vi "Register gRPC Methods.vi"(8 "error in (no error)":errorcluster, 11 "Template Server in":refnum<class "MicronGRPC.lvclass">) -> (0 "error out":errorcluster, 3 "Template Server out":refnum<class "MicronGRPC.lvclass">)   [LabVIEW 2019, in "MicronGRPCGeneratedServer.lvlib" / "MicronGRPC.lvclass"]
uses:
  MicronGRPC.lvclass
  typeDefs/Server Internal UEs.ctl
  typeDefs/Server Internal Message.ctl
  typeDefs/Server gRPC UEs.ctl
  <vilib>/gRPC/LabVIEW gRPC Library/Server API/typeDefs/gRPCId Cluster.ctl
  <vilib>/gRPC/LabVIEW gRPC Library/Shared/grpcId.ctl
  MicronGRPC.lvclass/MicronGRPC.ctl
  <vilib>/gRPC/LabVIEW gRPC Library/grpc-lvsupport-release.lvlib
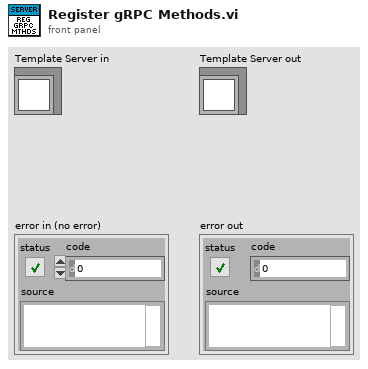
[diagram p1: front panel]
types:
  T1 = typedef "MicronGRPCGeneratedServer.lvlib/MicronGRPC.lvclass/Server gRPC UEs.ctl" = cluster{"MicronGRPC Message gRPC UE":refnum<user-event>}
  T2 = typedef "MicronGRPCGeneratedServer.lvlib/MicronGRPC.lvclass/Server Internal UEs.ctl" = cluster{"MicronGRPC Message Internal UE":refnum<user-event>}
  T3 = typedef "grpc-lvsupport-release.lvlib/grpcId.ctl" = u64
  T4 = typedef "MicronGRPCGeneratedServer.lvlib/MicronGRPC.lvclass/Server Internal Message UE.ctl" = refnum<user-event>
  T5 = typedef "grpc-lvsupport-release.lvlib/gRPCId Cluster UE.ctl" = refnum<user-event>
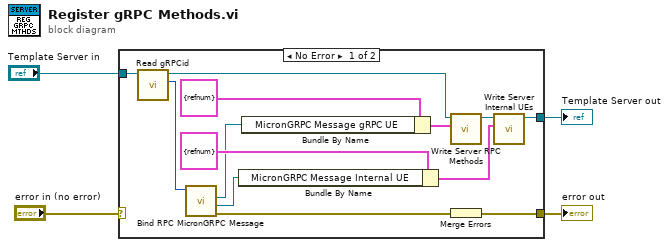
[diagram p0: block diagram]
diagram:
  n1 = case shown="No Error" "error in (no error)" {
    selector: "error in (no error)" -> [_ w18]
    tunnel: "Template Server in" -> [w9 w19]
    tunnel: [w17 w18] -> w3
    tunnel: [w16 w19] -> w2
    frame No Error {
      n2 = call-dynamic "Read gRPCid.vi"("gRPC service in"=w9) -> ("gRPCid"=w8:T3, "gRPC service out"=w10:refnum<class "MicronGRPC.lvclass">)  [unwired: 8 in, 1 out]
      n3 = call "Bind RPC MicronGRPC Message.vi"("gRPCid server in"=w8) -> ("error out"=w7:errorcluster, "MicronGRPC Message Internal UE"=w6:T4, "MicronGRPC Message gRPC UE"=w5:T5)  [unwired: 7 in, 1 out]
      n4 = Bundle By Name ("Bundle Internal UEs")(cluster=T2 {"MicronGRPC Message Internal UE"=refnum} ("Server Internal UEs"), "MicronGRPC Message Internal UE"=w6) -> (w15:T2)
      n5 = Bundle By Name ("Bundle gRPC UEs")(cluster=T1 {"MicronGRPC Message gRPC UE"=refnum} ("gRPC Server Method Events"), "MicronGRPC Message gRPC UE"=w5) -> (w12:T1)
      n6 = call "Write Server RPC Methods.vi"("Server RPC Methods"=w12, "SignalGeneratorService in"=w10) -> ("SignalGeneratorService out"=w13:refnum<class "MicronGRPC.lvclass">)  [unwired: 8 in, 1 out]
      n7 = Merge Errors(w7) -> (w17:errorcluster)
      n8 = call "Write Server Internal UEs.vi"("Server Internal UEs"=w15, "SignalGeneratorService in"=w13) -> ("SignalGeneratorService out"=w16:refnum<class "MicronGRPC.lvclass">)  [unwired: 8 in, 1 out]
    }
    frame Error {
    }
  }
  "error out" <- w3
  "Template Server out" <- w2
